vi "Decouple 5-bar Mechanism.vi"(2 "5-bar Side":T1, 3 "motors angles":dbl[](array[numeric])=[0.0, 0.0, 0.0, 0.0, 0.0, 0.0, 0.0]) -> (0 "joint angles":dbl[](array[numeric]))   [LabVIEW 2011, in "Finger.lvclass"]
uses:
  Finger.lvclass
  Controls/5-bar Side.ctl
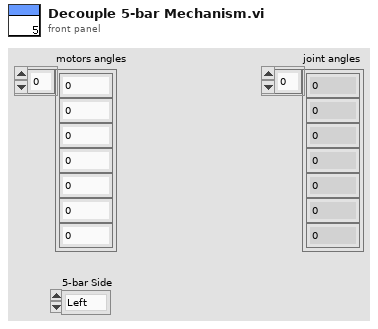
[diagram p1: front panel]
types:
  T1 = typedef "5-bar Side.ctl" = enum16{"Left", "Right"}
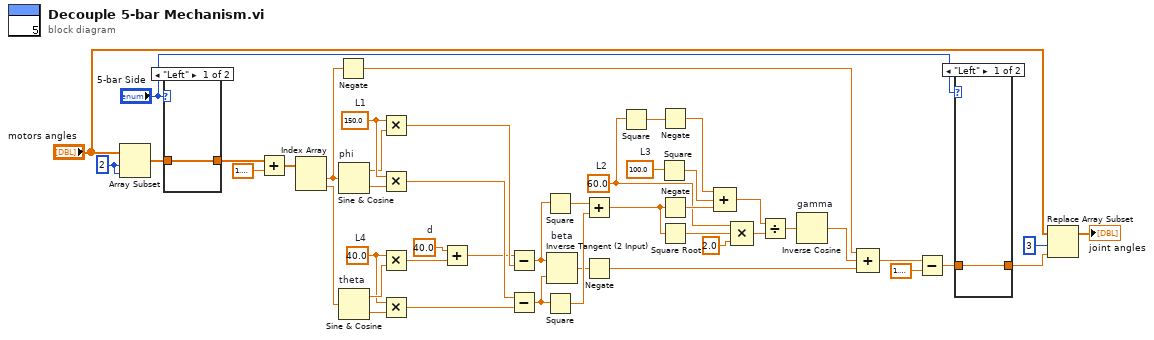
[diagram p0: block diagram]
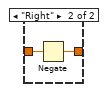
[diagram p2: hidden frame]
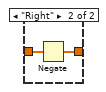
[diagram p3: hidden frame]
diagram:
  w10 = 40.0  # d
  w29 = 100.0  # L3
  w24 = 60.0  # L2
  w46 = 2 ("index")
  w43 = 40.0  # L4
  w41 = 150.0  # L1
  n1 = Array Subset(array="motors angles", index=w46, length=w46) -> (w2:dbl[])
  n2 = case shown="\"Left\"" "5-bar Side" {
    tunnel: w2 -> [w48 w50]
    tunnel: [w48 w49] -> w1
    frame "Left" {
    }
    frame "Right" {
      n3 = Negate(x=w50) -> (-x=w49:dbl[])
    }
  }
  n4 = Add(x=w1, y=1.5707963267948966) -> (x+y=w3:dbl[])
  n5 = Index Array(array=w3) -> (element #1=w20:dbl, element #2=w45:dbl)  [unwired: 2 in]
  n6 = Negate(x=w20) -> (-x=w21:dbl)
  n7 = Sine & Cosine "phi"(0:w20) -> (1:w40:dbl, 2:w39:dbl)
  n8 = Sine & Cosine "theta"(0:w45) -> (1:w44:dbl, 2:w42:dbl)
  n9 = Multiply(x=w41, y=w40) -> (x*y=w12:dbl)
  n10 = Multiply(x=w41, y=w39) -> (x*y=w37:dbl)
  n11 = Multiply(x=w43, y=w44) -> (x*y=w11:dbl)
  n12 = Multiply(x=w43, y=w42) -> (x*y=w38:dbl)
  n13 = Add(x=w10, y=w11) -> (x+y=w9:dbl)
  n14 = Subtract(x=w9, y=w12) -> (x-y=w14:dbl)
  n15 = Subtract(x=w37, y=w38) -> (x-y=w13:dbl)
  n16 = Square(x=w14) -> (x^2=w36:dbl)
  n17 = Square(x=w13) -> (x^2=w35:dbl)
  n18 = Inverse Tangent (2 Input) "beta"(1:w13, 2:w14) -> (0:w22:dbl)
  n19 = Add(x=w36, y=w35) -> (x+y=w31:dbl)
  n20 = Negate(x=w22) -> (-x=w18:dbl)
  n21 = Square(x=w24) -> (x^2=w33:dbl)
  n22 = Square(x=w29) -> (x^2=w25:dbl)
  n23 = Negate(x=w33) -> (-x=w26:dbl)
  n24 = Negate(x=w31) -> (-x=w34:dbl)
  n25 = Square Root(x=w31) -> (sqrt(x)=w30:dbl)
  n26 = Compound Arithmetic op=ADD(w26, w25, w34) -> (w32:dbl)
  n27 = Compound Arithmetic op=MULTIPLY(w24, w30, 2.0 ("value")) -> (w27:dbl)
  n28 = Divide(x=w32, y=w27) -> (x/y=w23:dbl)
  n29 = Inverse Cosine "gamma"(1:w23) -> (0:w19:dbl)
  n30 = Compound Arithmetic op=ADD(w21, w19, w18) -> (w6:dbl)
  n31 = Subtract(x=w6, y=1.5707963267948966) -> (x-y=w4:dbl)
  n32 = case shown="\"Left\"" "5-bar Side" {
    tunnel: w4 -> [w51 w53]
    tunnel: [w51 w52] -> w8
    frame "Left" {
    }
    frame "Right" {
      n33 = Negate(x=w53) -> (-x=w52:dbl)
    }
  }
  n34 = Replace Array Subset(array="motors angles", new element=w8, index=3) -> (→"joint angles":dbl[])
